vi "Find Control Ref 2D.vi"(10 "Ctl Refnum":refnum<vi>, 11 "2D Array":refnum<vi>[][](array[refnum])) -> (2 "Index":i32, 3 "MUX Selection":T1)   [LabVIEW 2022 SP3, in "TouchControl.lvlib" / "MuxPanel.lvclass"]
uses:
  MuxPanel.lvclass
  MuxPanel.lvclass/MuxPanel.ctl
  MUX Selection.ctl
  TouchControl.lvlib
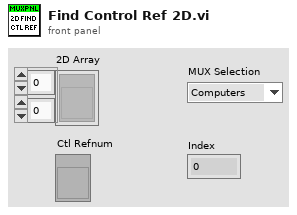
[diagram p1: front panel]
types:
  T1 = typedef "TouchControl.lvlib/MUX Selection.ctl" = enum16{"Computers", "Others"}
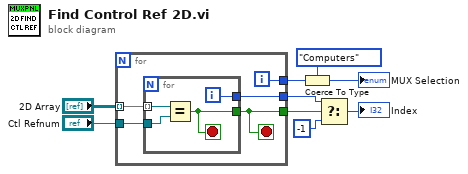
[diagram p0: block diagram]
diagram:
  n1 = for {
    tunnel: "2D Array" -> [w14] mode=indexing
    tunnel: "Ctl Refnum" -> [w13]
    tunnel: [w12] -> w4
    tunnel: [w11] -> w3
    tunnel: [w10] -> w7
    i -> [w10]
    stop <- w12 stop-if-true
    n2 = for {
      tunnel: w14 -> [w18] mode=indexing
      tunnel: w13 -> [w17]
      tunnel: [w16] -> w12
      tunnel: [w15] -> w11
      i -> [w15]
      stop <- w16 stop-if-true
      n3 = Equal?(x=w18, y=w17) -> (x = y?=w16:bool)
    }
  }
  n4 = Coerce To Type(0:w7, 1:MUX_Selection."Computers" ("MUX Selection")) -> (2:→"MUX Selection":T1)
  n5 = Select(t=w3, s=w4, f=-1) -> (s? t:f=→"Index":i32)
